vi "Eth Status Write Write Enable.vi"(7 "Status Reference":T1, 8 "error in (no error)":errorcluster, 9 "Write Enable":bool, 11 "N":i32) -> (0 "error out":errorcluster)   [LabVIEW 2019, in "Eth Status.lvlib"]
uses:
  Eth Status.lvlib
  Ctl/ICPCON Status.ctl
  MB_TCP2/MB_TCP_State.ctl
  MB_TCP2/MB_TCP.lvclass
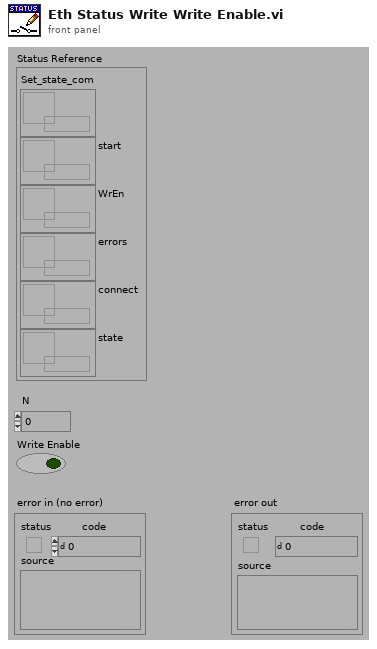
[diagram p1: front panel]
types:
  T1 = typedef "Eth Status.lvlib/ICPCON Status.ctl" = cluster{"Set_state_com":refnum<data-value>, "start":refnum<data-value>, "WrEn":refnum<data-value>, "errors":refnum<data-value>, "connect":refnum<data-value>, "state":refnum<data-value>}
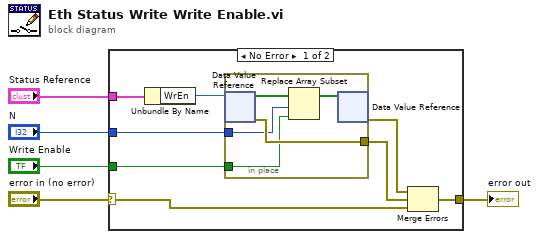
[diagram p0: block diagram]
diagram:
  n1 = case shown="No Error" "error in (no error)" {
    selector: "error in (no error)" -> [w6 w19]
    tunnel: [w11 w19] -> w4
    tunnel: "N" -> [w13 _]
    tunnel: "Status Reference" -> [w12 _]
    tunnel: "Write Enable" -> [w10 _]
    frame No Error {
      n2 = Unbundle By Name(w12) -> ("WrEn"=w7:refnum<data-value>)
      n3 = in-place {
        in-place-border: w13 -> [w15]
        in-place-border: [w18] -> w8
        in-place-border: w10 -> [w14]
        n4 = in-place-dvr #1(w7) -> (w17:bool[], w18:errorcluster)
        n5 = Replace Array Subset(array=w17, new element=w14, index=w15) -> (w16:bool[])
        n6 = in-place-dvr #1(w16) -> (w9:errorcluster)  [unwired: 1 out]
      }
      n7 = Merge Errors(w9, w8, w6) -> (w11:errorcluster)
    }
    frame Error {
    }
  }
  "error out" <- w4
